vi "GPIO Write.vi"(8 "error in (no error)":errorcluster, 9 "Output Value":bool, 10 "DO Channel":u8, 11 "LINX GPIO in":refnum<class "LINX GPIO.lvclass">) -> (0 "error out":errorcluster, 3 "LINX GPIO out":refnum<class "LINX GPIO.lvclass">)   [LabVIEW 2020, in "LINX GPIO.lvclass"]
doc: "Enables/disables the specified GPIO channel."
uses:
  LINX GPIO.lvclass
  LINX GPIO.lvclass/LINX GPIO.ctl
  <vilib>/MakerHub/LINX/Public/Peripherals/Digital/Digital Write 1 Chan.vi
  <vilib>/MakerHub/LINX/Public/Peripherals/Digital/Digital Write N Chans.vi
  <vilib>/MakerHub/LINX/Private/Local IO/LinxDigitalWrite.vi
  <vilib>/MakerHub/LINX/Public/Utilities/Check Channel.vi
  <vilib>/MakerHub/LINX/Private/Local IO/Handle Errors.vi
  <vilib>/MakerHub/LINX/Private/Utilties/Generate Error.vi
  <vilib>/MakerHub/LINX/LMH-LINX.lvlib
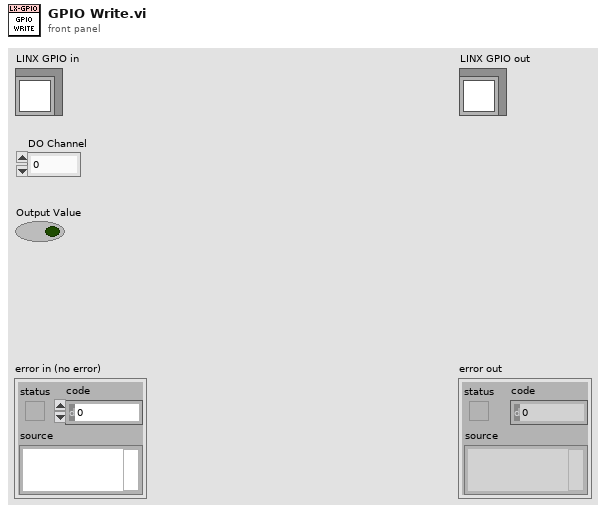
[diagram p1: front panel]
types:
  T1 = typedef "LMH-LINX.lvlib/LINX Ref.ctl" = cluster{"IO":T2, "Interface":T3, "LINX Device Config":T4}
  T2 = typedef "LMH-LINX.lvlib/Platform.ctl" = enum16{"Remote", "Local"}
  T3 = typedef "LMH-LINX.lvlib/Interface.ctl" = enum16{"Serial", "TCP"}
  T4 = typedef "LMH-LINX.lvlib/Device.lvlib/LINX Device Config.ctl" = cluster{"Interface":T3, "COM Port":refnum<visa-resource-name>, "TCP Configuration":T5, "Device Family":u8, "Device ID":u8, "Device Name":string, "TCP Ref":refnum<k5>, "Channels":T6}
  T5 = typedef "LMH-LINX.lvlib/Device.lvlib/TCP Config.ctl" = cluster{"IP Address":string, "Port":u16}
  T6 = typedef "LMH-LINX.lvlib/Channels.ctl" = cluster{"DI":u8[], "DO":u8[], "AI":u8[], "AO":u8[], "PWM":u8[], "QE":u8[], "UART":u8[], "I2C 2":u8[], "SPI":u8[], "CAN":u8[], "Servo":u8[], "AI Ref (V)":dbl, "AI Resolution (Bits)":u8, "AO Ref (V)":dbl, "AO Resolution (Bits)":u8}
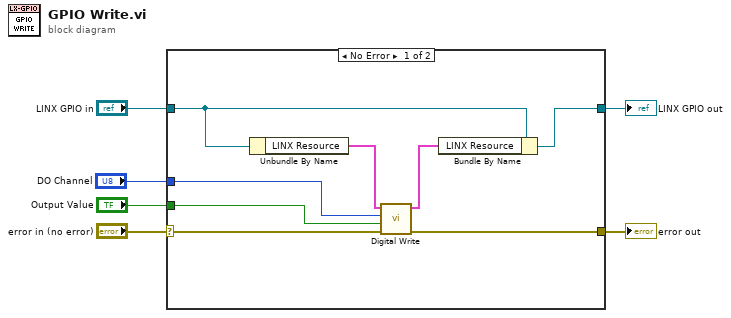
[diagram p0: block diagram]
diagram:
  n1 = case shown="No Error" "error in (no error)" {
    selector: "error in (no error)" -> [w10 w16]
    tunnel: [w9 w16] -> w5
    tunnel: [w12 w15] -> w3
    tunnel: "LINX GPIO in" -> [w13 w15]
    tunnel: "Output Value" -> [w8 _]
    tunnel: "DO Channel" -> [w7 _]
    frame No Error {
      n2 = Unbundle By Name(w13) -> ("LINX Resource"=w14:T1)
      n3 = call-poly <vilib>:"Digital Write.vi"("Error In"=w10, "Output Value"=w8, "DO Channel"=w7, "LINX Resource"=w14) -> ("Error Out"=w9:errorcluster, "LINX Resource"=w11:T1)  [unwired: 6 in]
      n4 = Bundle By Name(cluster=w13, "LINX Resource"=w11) -> (w12:refnum<class "LINX GPIO.lvclass">)
    }
    frame Error {
    }
  }
  "error out" <- w5
  "LINX GPIO out" <- w3
